vi "chaos crest update.vi"(7 "data":u32, 9 "attr_pos":i32, 10 "cu_uid":u32, 11 "h":u32) -> (2 "function return":i32, 3 "h out":u32, 5 "data out":u32)   [LabVIEW 2014, in "libcommon-crest.lvlib"]
doc: "int chaos_crest_update(chaos_crest_handle_t h,uint32_t cu_uid,int attr_pos,void*data);"
uses:
  libcommon-crest.lvlib
  chaos-i686-dynamic-release/lib/libcommon-crest.so
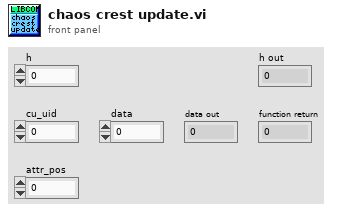
[diagram p1: front panel]
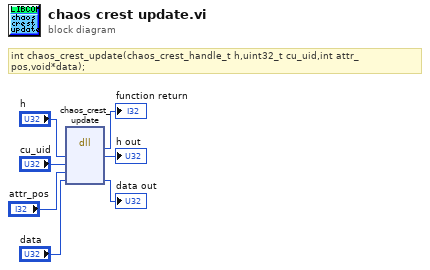
[diagram p0: block diagram]
diagram:
  # "int chaos_crest_update(chaos_crest_handle_t h,uint32_t cu_uid,int attr_pos,void*data);"
  n1 = dll-call lib="home/chaos/chaos_bundle/chaos-i686-dynamic-release/lib/libcommon-crest.*" fn="chaos_crest_update"("h"="h", "cu_uid"="cu_uid", "attr_pos"="attr_pos", "data"="data") -> (→"function return":i32, "h"=→"h out":u32, "data"=→"data out":u32)  [unwired: 5 in, 2 out]
